vi "Destruct.vi"(8 "error in (no error)":errorcluster, 11 "muExpr in":refnum<class "mupExpr.lvclass">) -> (0 "error out":errorcluster)   [LabVIEW 2015, in "mupExpr.lvclass"]
doc: "Destruct the muExpr instance. This will release the muParser handle and variable pointers."
uses:
  mupExpr.lvclass
  mupExpr.lvclass/mupExpr.ctl
  mupLib/mupLibPath.vi
  mupLib/mupLib.lvlib
panel:
  # "Destruct the muExpr instance. This will release the muParser handle and variable pointers."
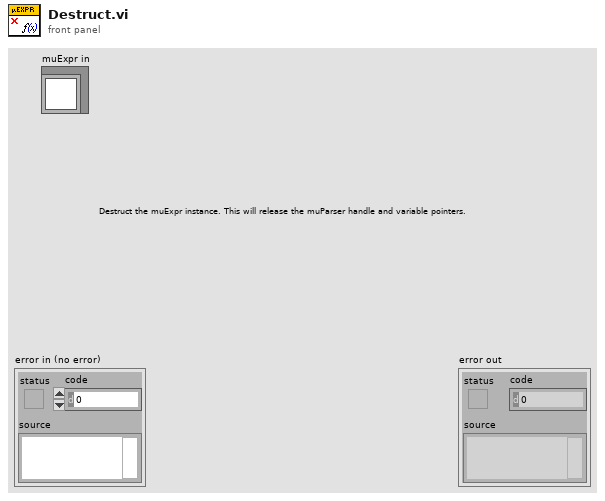
[diagram p1: front panel]
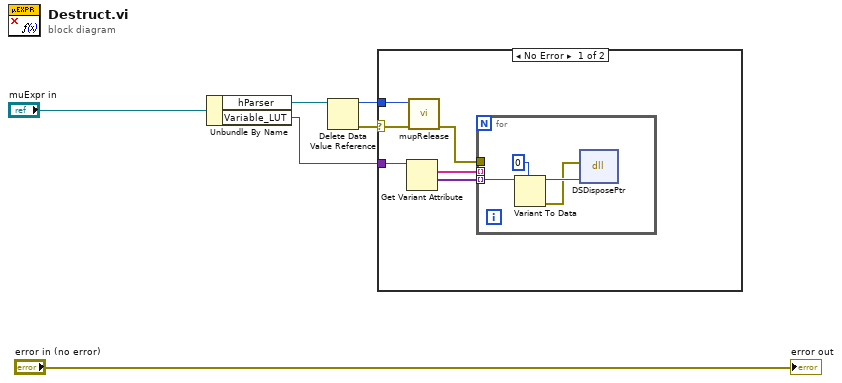
[diagram p0: block diagram]
diagram:
  n1 = Unbundle By Name("muExpr in") -> ("hParser"=w3:refnum<data-value>, "Variable_LUT"=w4:variant)
  n2 = Delete Data Value Reference(data value reference=w3) -> (data value=w2:u64, error out=w1:errorcluster)  [unwired: 1 in]
  n3 = case shown="No Error" w1 {
    selector: w1 -> [w7 _]
    tunnel: w4 -> [w12 _]
    tunnel: w2 -> [w8 _]
    frame No Error {
      n4 = Get Variant Attribute(Variant=w12) -> (names=w11:string[], values=w9:variant[])  [unwired: 3 in, 2 out]
      n5 = call "mupRelease.vi"("error in (no error)"=w7, "hParser in"=w8) -> ("error out"=w10:errorcluster)  [unwired: 9 in]
      n6 = for {
        tunnel: w11 -> [_] mode=indexing
        tunnel: w10 -> [_]
        tunnel: w9 -> [w16] mode=indexing
        n7 = Variant To Data(type=u64 0, Variant=w16) -> (data=w14:u64, error out=w13:errorcluster)  [unwired: 1 in]
        n8 = dll-call lib="LabVIEW" fn="DSDisposePtr"(error in=w13, "ptr"=w14) -> ()  [unwired: 4 in, 2 out]
      }
    }
    frame Error {
    }
  }
  "error out" <- "error in (no error)"
